vi "Get Status Error Channel Data References.vi"(8 "error in":errorcluster, 11 "custom device ref in":T1 format="%.0x") -> (0 "error out":errorcluster, 1 "status channel data references":T3 {"receiving" format="%.0x"; "specific errors"."gap" format="%.0x"; "specific errors"."parity" format="%.0x"; "specific errors"."long word" format="%.0x"; "specific errors"."bit timing" format="%.0x"; "specific errors"."timeout" format="%.0x"}, 3 "custom device ref out":T1 format="%.0x")   [LabVIEW 2020]
uses:
  Scripting/Ballard ARINC 429 Scripting.lvlib
  <vilib>/NI VeriStand/Custom Device API/Custom Device API.lvlib
  <vilib>/NI VeriStand/Custom Device API/Data Reference.ctl
  <vilib>/NI VeriStand/Custom Device API/Data Access Type.ctl
  <vilib>/NI VeriStand/Custom Device API/Custom Device Item Ref.ctl
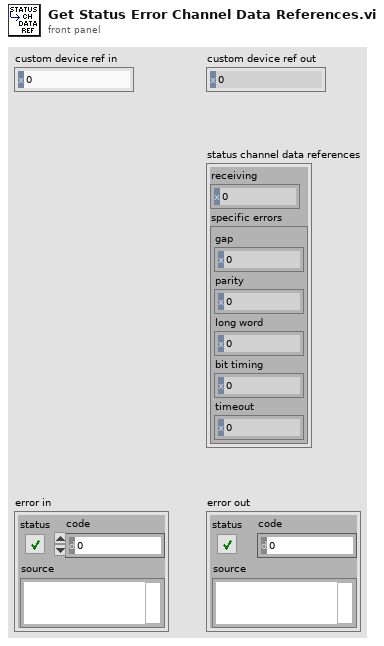
[diagram p1: front panel]
types:
  T1 = typedef "Custom Device API.lvlib/Custom Device Item Ref.ctl" = u64
  T2 = typedef "Custom Device API.lvlib/Data Reference.ctl" = i32
  T3 = cluster{"receiving":T2, "specific errors":cluster{"gap":T2, "parity":T2, "long word ":T2, "bit timing":T2, "timeout":T2}}
  T4 = typedef "Custom Device API.lvlib/Data Access Type.ctl" = enum16{"Read", "Write"}
  T5 = cluster{"gap":T1, "parity":T1, "long word":T1, "bit timing":T1, "timeout":T1}
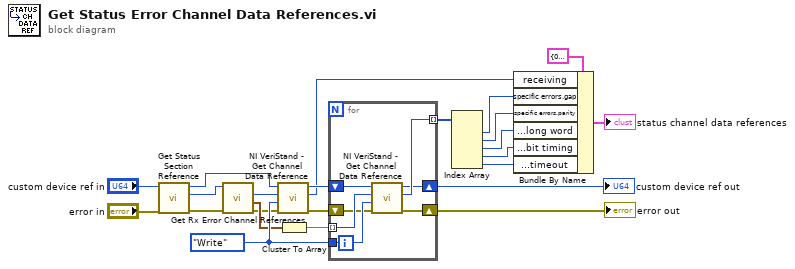
[diagram p0: block diagram]
diagram:
  w17 = Data_Access_Type."Write" ("Access")
  n1 = call "Get Status Section Reference.vi"("error in"="error in", "Ballard ARINC 429 ref"="custom device ref in") -> ("error out"=w21:errorcluster, "status section reference"=w22:T1, "Ballard ARINC 429 ref out"=w2:T1)  [unwired: 7 in]
  n2 = call "Get Rx Error Channel References.vi"("error in"=w21, "status reference in"=w22) -> ("error out"=w14:errorcluster, "Rx specific error count references"=w15:T5, "Rx error count reference"=w18:T1)  [unwired: 6 in, 1 out]
  n3 = call <vilib>:"NI VeriStand - Get Channel Data Reference.vi"("error in (no error)"=w14, "Access"=w17, "Channel Ref in"=w18, "Device Ref in"=w2) -> ("error out"=w12:errorcluster, "Channel Data Reference"=w5:T2, "Device Ref out"=w16:T1)  [unwired: 5 in]
  n4 = Cluster To Array(cluster=w15) -> (array=w13:T1[])
  n5 = for {
    tunnel: w17 -> [w30]
    tunnel: w13 -> [w28] mode=indexing
    tunnel: [w26] -> w11 mode=indexing
    shift-right: [w25] -> w4
    shift-left: w12 -> [w27]
    shift-right: [w24] -> w1
    shift-left: w16 -> [w29]
    n6 = call <vilib>:"NI VeriStand - Get Channel Data Reference.vi"("error in (no error)"=w27, "Access"=w30, "Channel Ref in"=w28, "Device Ref in"=w29) -> ("error out"=w25:errorcluster, "Channel Data Reference"=w26:T2, "Device Ref out"=w24:T1)  [unwired: 5 in]
  }
  "error out" <- w4
  "custom device ref out" <- w1
  n7 = Index Array(array=w11) -> (element #1=w10:T2, element #2=w9:T2, element #3=w8:T2, element #4=w7:T2, element #5=w6:T2)  [unwired: 5 in]
  n8 = Bundle By Name(cluster=T3 {"receiving"=0, "specific errors"={"gap"=0, "parity"=0, "long word "=0, "bit timing"=0, "timeout"=0}} ("status error channel data references"), "receiving"=w5, "specific errors.gap"=w10, "specific errors.parity"=w9, "specific errors.long word"=w8, "specific errors.bit timing"=w7, "specific errors.timeout"=w6) -> (→"status channel data references":T3)
